vi "File Reader.vi"(0 "XML File Path":path, 11 "error in":errorcluster) -> (4 "Velocity Profiles":dbl[][][](array[numeric]), 6 "Intermediate Headings":dbl[](array[numeric]), 8 "Position Command Groups":T2(array[cluster]), 10 "Time Command Groups":T1(array[cluster]), 14 "Delta Time":dbl, 15 "error out":errorcluster)   [LabVIEW 2015]
uses:
  <vilib>/regexp/Match Regular Expression.xnode
panel:
  out "Play":string[](array[string])
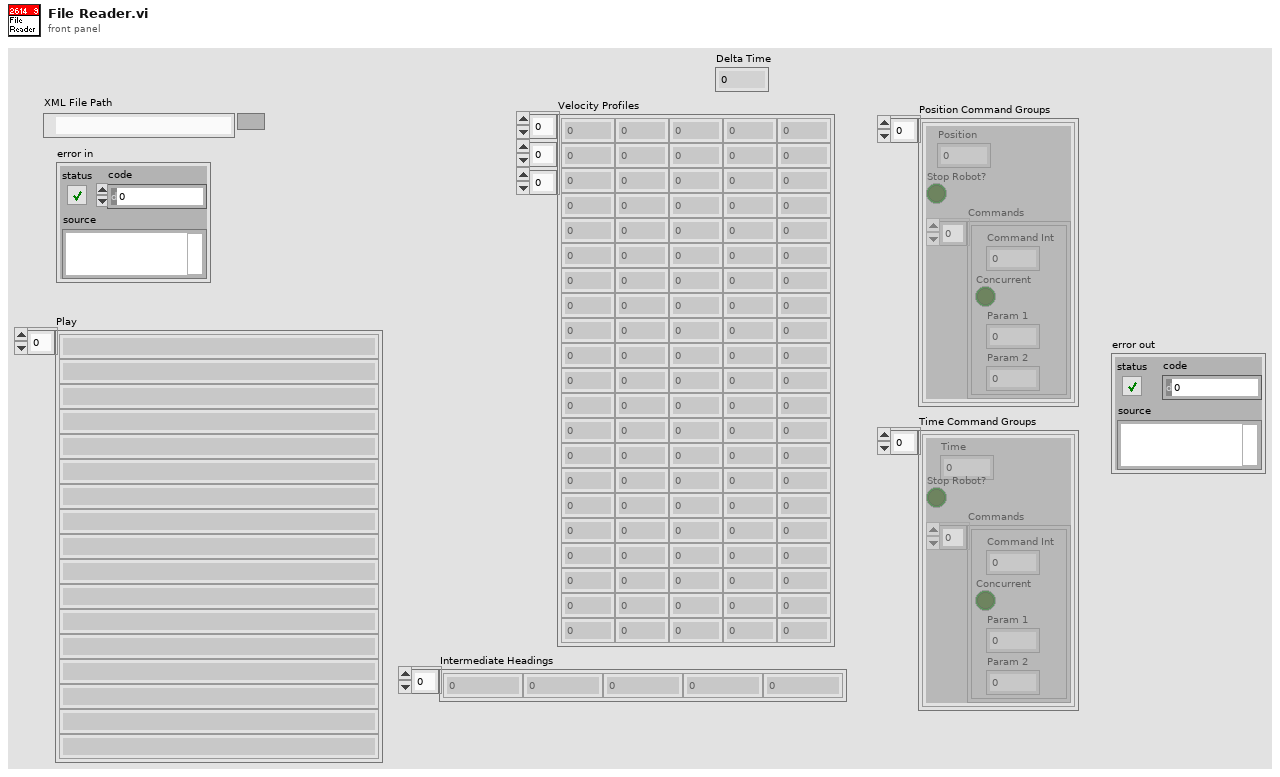
[diagram p1: front panel]
types:
  T1 = cluster{"Stop Robot?":bool, "Commands":cluster{"Command Int":i32, "Concurrent":bool, "Param 1":dbl, "Param 2":dbl}[], "Time":dbl}[]
  T2 = cluster{"Position":i32, "Stop Robot?":bool, "Commands":cluster{"Command Int":i32, "Concurrent":bool, "Param 1":dbl, "Param 2":dbl}[]}[]
  T3 = cluster{"Command Int":i32, "Concurrent":bool, "Param 1":dbl, "Param 2":dbl}[]
  T4 = cluster{"Position":i32, "Stop Robot?":bool, "Commands":cluster{"Command Int":i32, "Concurrent":bool, "Param 1":dbl, "Param 2":dbl}[]}
  T5 = cluster{"Command Int":i32, "Concurrent":bool, "Param 1":dbl, "Param 2":dbl}
  T6 = cluster{"Stop Robot?":bool, "Commands":cluster{"Command Int":i32, "Concurrent":bool, "Param 1":dbl, "Param 2":dbl}[], "Time":dbl}
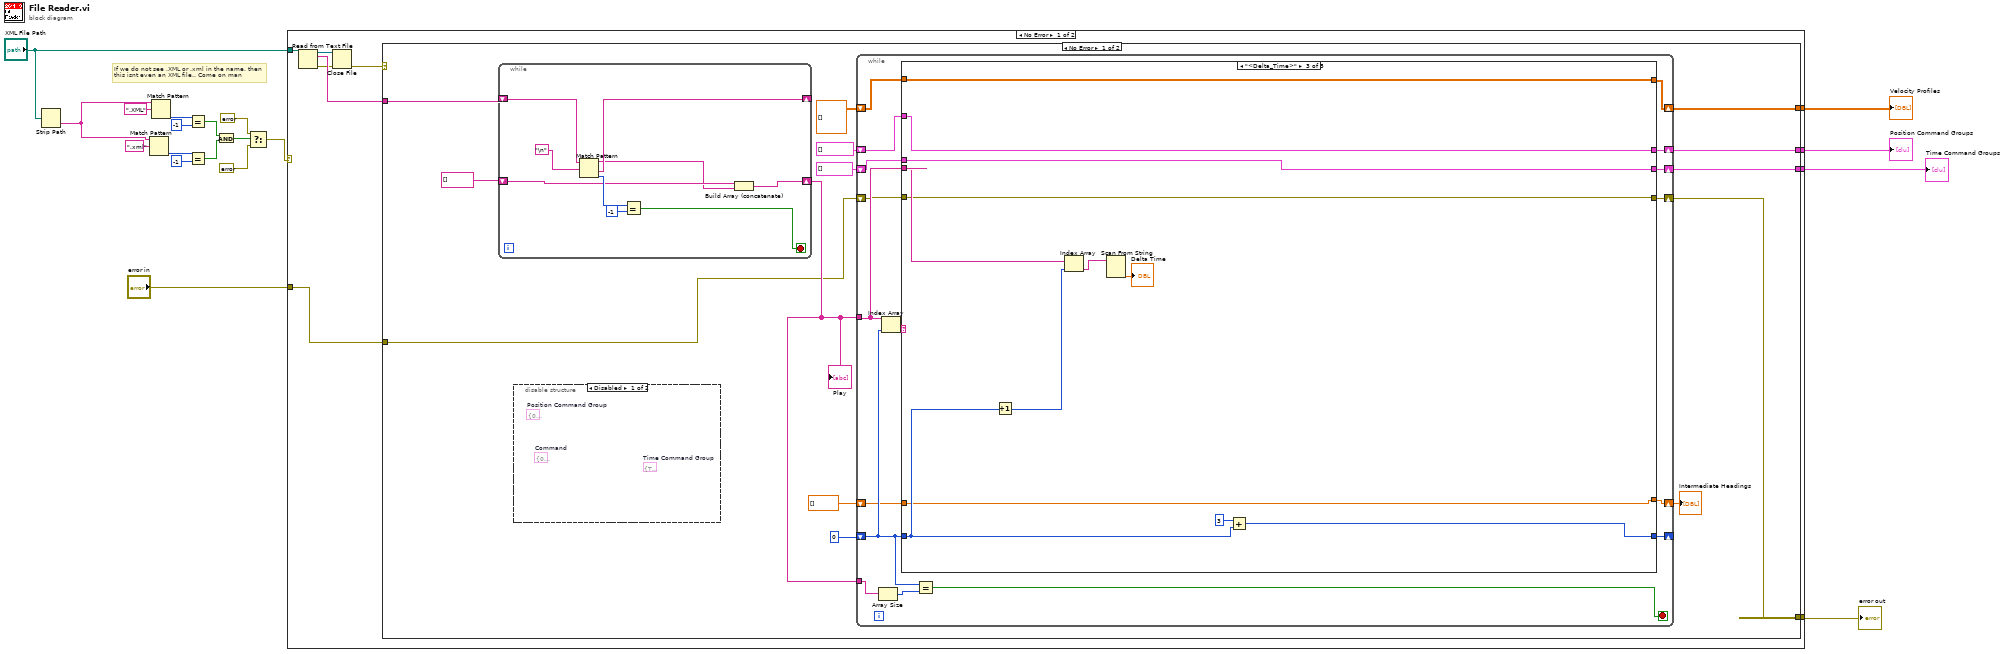
[diagram p0: block diagram]
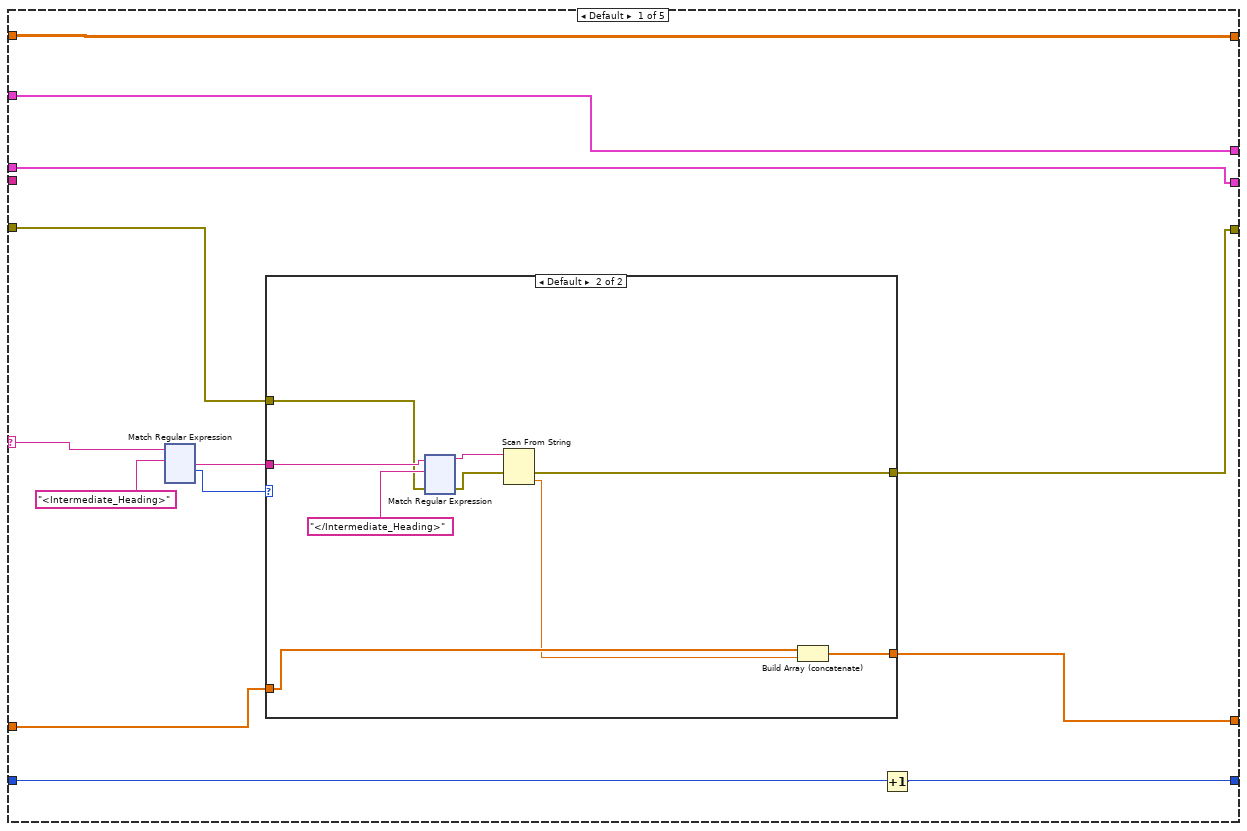
[diagram p3: hidden frame]
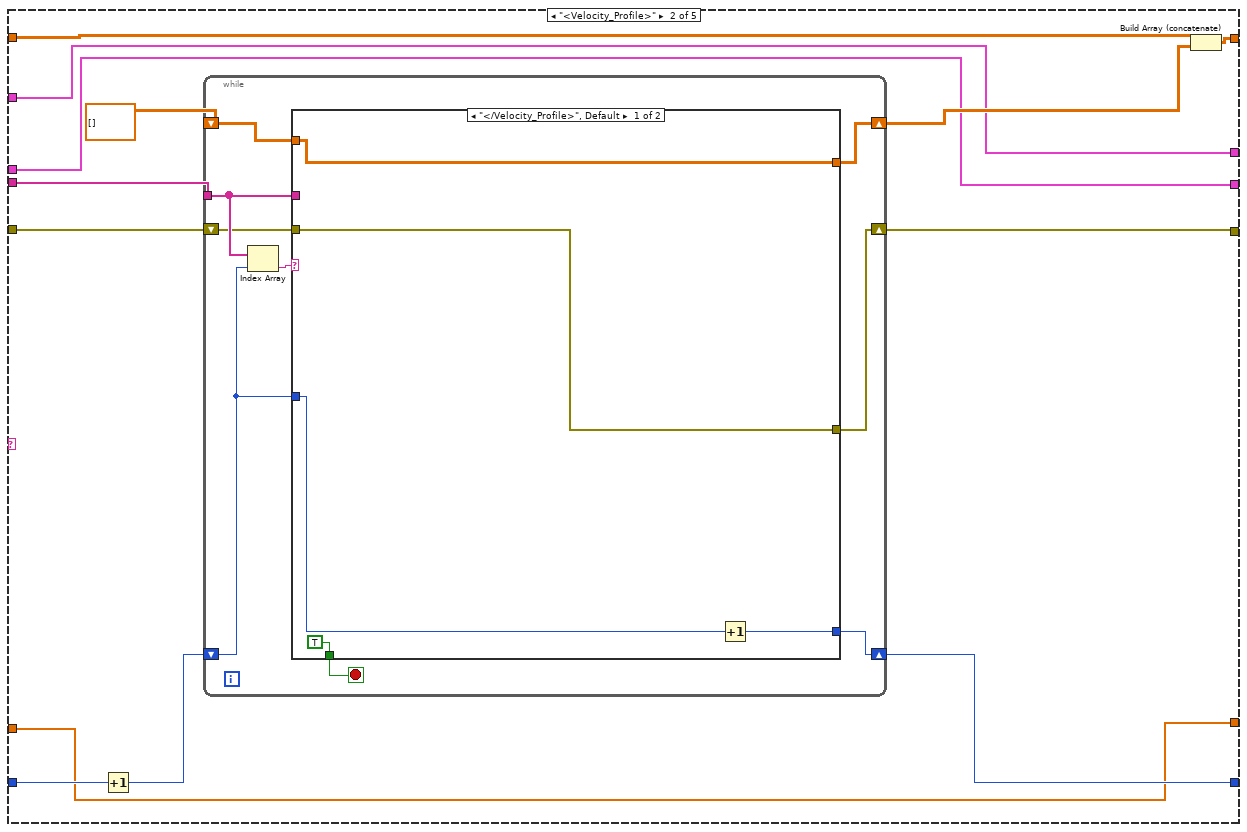
[diagram p5: hidden frame]
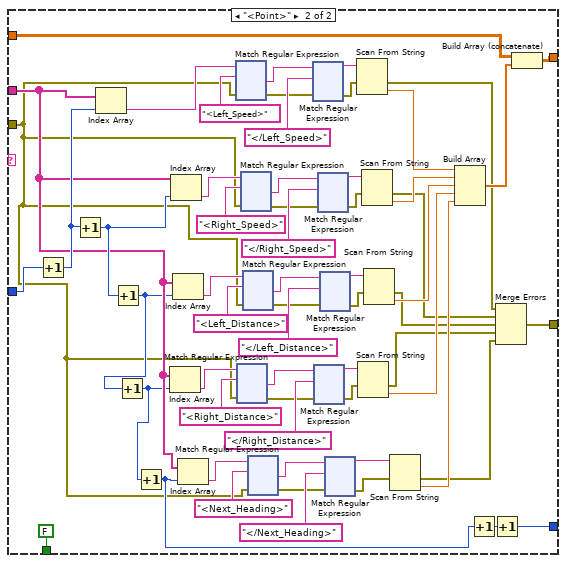
[diagram p6: hidden frame]
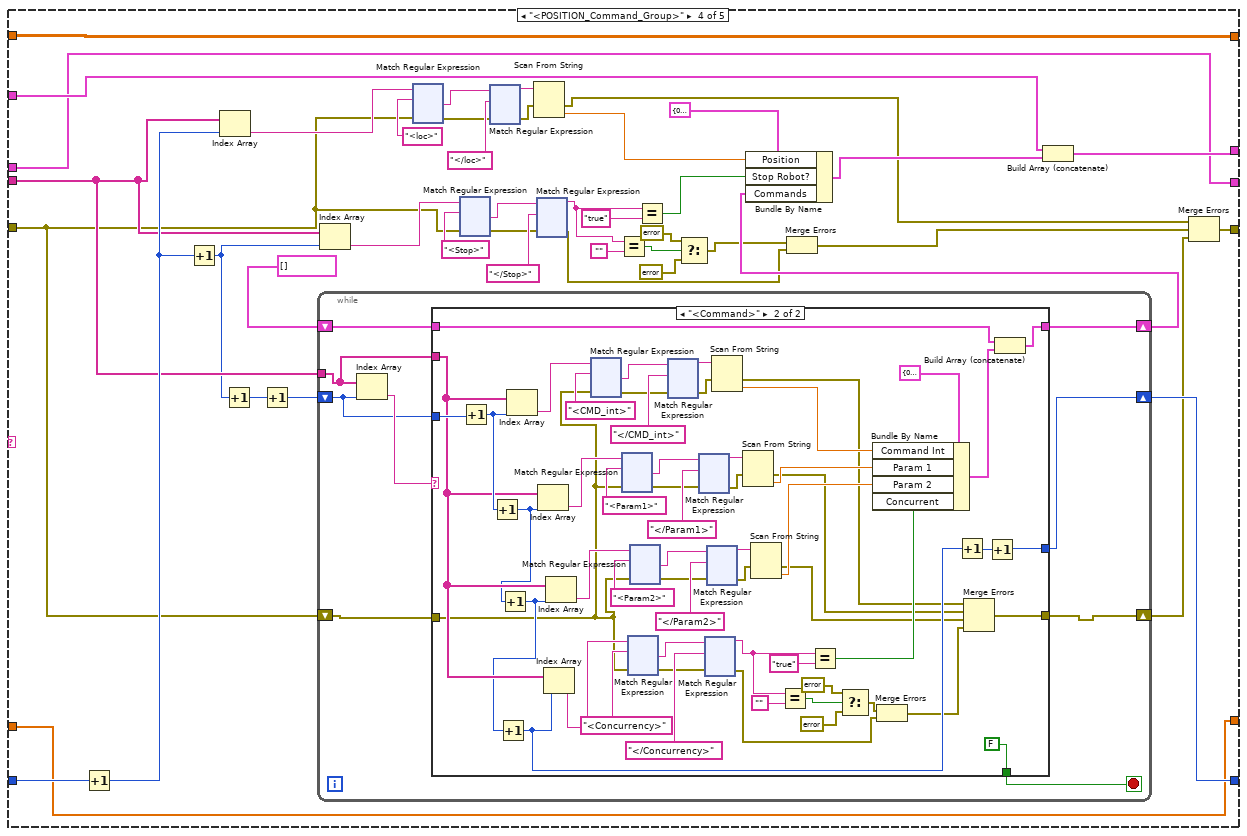
[diagram p7: hidden frame]
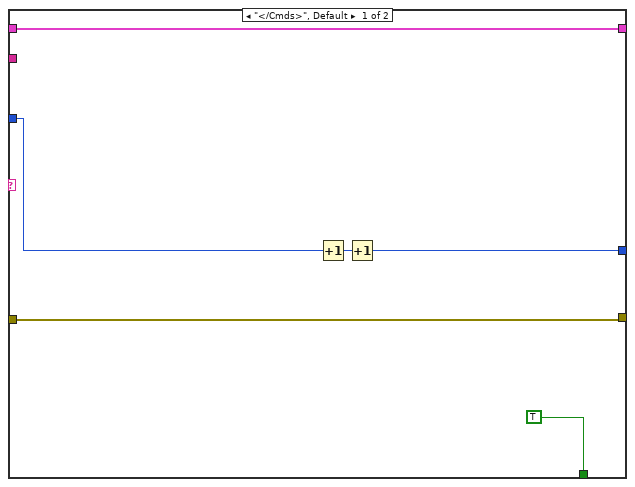
[diagram p8: hidden frame]
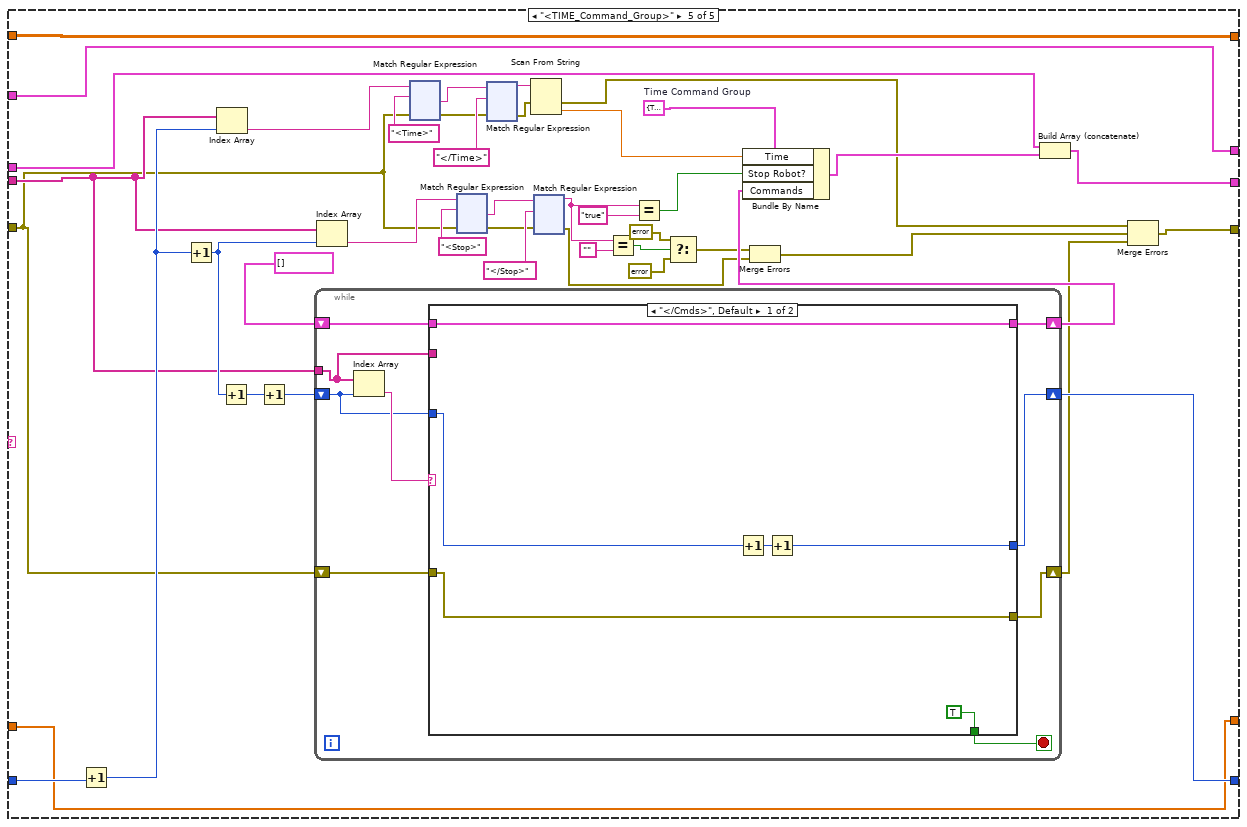
[diagram p9: hidden frame]
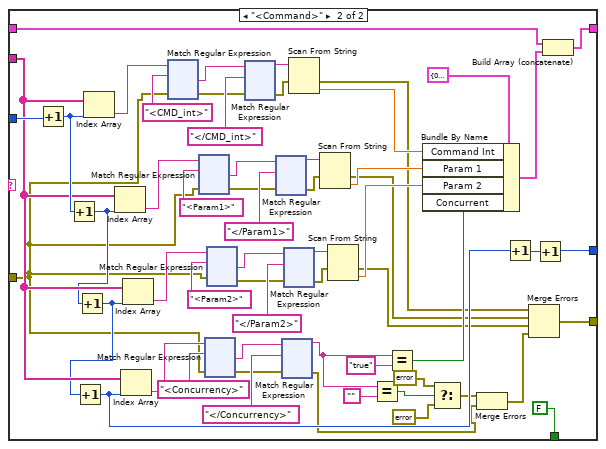
[diagram p10: hidden frame]
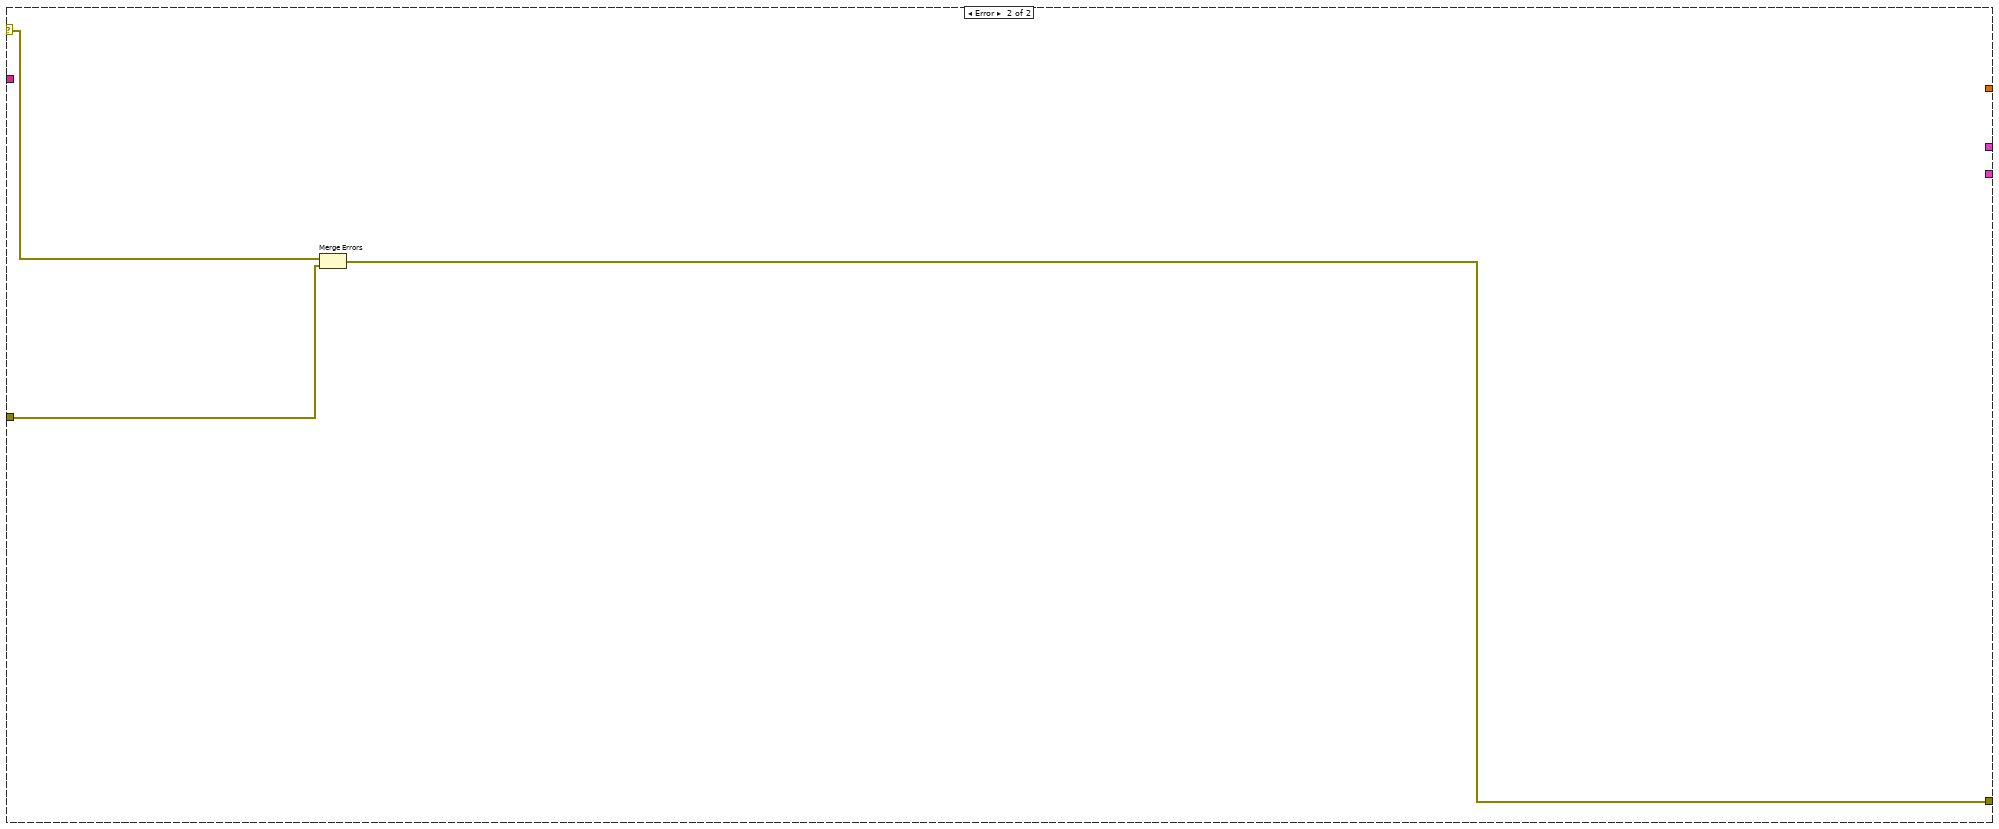
[diagram p11: hidden frame]
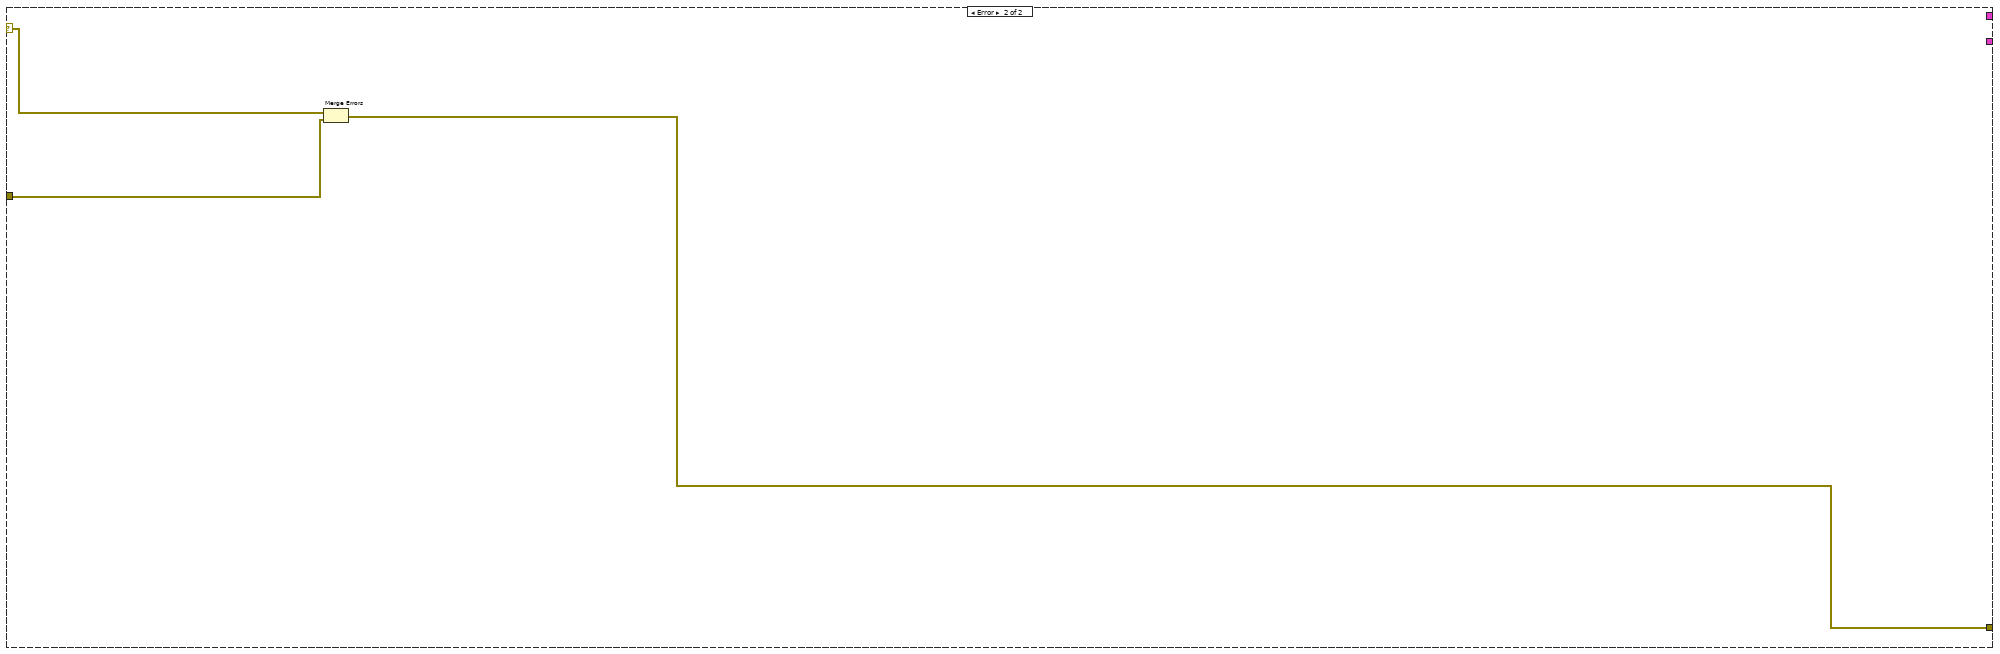
[diagram p12: hidden frame]
diagram:
  # "If we do not see .XML or .xml in the name. then\nthis isnt even an XML file.. Come on man"
  n1 = Strip Path(path="XML File Path") -> (name=w17:string)  [unwired: 1 out]
  n2 = Match Pattern(string=w17, regular expression=".xml") -> (offset past match=w13:i32)  [unwired: 1 in, 3 out]
  n3 = Match Pattern(string=w17, regular expression=".XML") -> (offset past match=w16:i32)  [unwired: 1 in, 3 out]
  n4 = Equal?(x=w16, y=-1) -> (x = y?=w12:bool)
  n5 = Equal?(x=w13, y=-1) -> (x = y?=w11:bool)
  n6 = And(x=w12, y=w11) -> (x .and. y?=w10:bool)
  n7 = Select(t=errorcluster {"status"=TRUE, "code"=13, "source"="File is not an XML File"} ("error in"), s=w10, f=errorcluster {"status"=FALSE, "code"=0, "source"=""} ("error in")) -> (s? t:f=w7:errorcluster)
  n8 = case shown="No Error" w7 {
    selector: w7 -> [_ w4532]
    tunnel: "XML File Path" -> [w29 _]
    tunnel: [w26 w4530] -> w5
    tunnel: "error in" -> [w27 w4531]
    tunnel: [w22 _] -> w3
    tunnel: [w21 _] -> w1
    tunnel: [w20 _] -> w2
    frame No Error {
      n9 = Read from Text File(file (use dialog)=w29) -> (refnum out=w24:refnum<file>, text=w28:string, error out=w25:errorcluster)  [unwired: 3 in, 1 out]
      n10 = Close File(refnum=w24, error in=w25) -> (error out=w23:errorcluster)  [unwired: 1 out]
      n11 = case shown="No Error" w23 {
        selector: w23 -> [_ w4529]
        tunnel: w28 -> [w43 _]
        tunnel: w27 -> [w34 w4528]
        tunnel: [w33 w4527] -> w26
        tunnel: [w32 _] -> w22
        tunnel: [w31 _] -> w21
        tunnel: [w30 _] -> w20
        frame No Error {
          n12 = while {
            shift-right: [w4525] -> _
            shift-left: w43 -> [w4526]
            shift-right: [w4524] -> w37
            shift-left: string[] [] -> [w4519]
            stop <- w4521 stop-if-true
            n13 = Match Pattern(string=w4526, regular expression="\n") -> (before substring=w4518:string, after substring=w4525:string, offset past match=w4523:i32)  [unwired: 1 in, 1 out]
            n14 = Equal?(x=w4523, y=-1) -> (x = y?=w4521:bool)
            n15 = Build Array (concatenate)(w4519, w4518) -> (w4524:string[])
          }
          "Play" <- w37
          n16 = disable-structure shown="Disabled" {
            frame Disabled {
              (unwired) T6 {"Stop Robot?"=TRUE, "Commands"=[], "Time"=0.0}  # Time Command Group
              (unwired) T5 {"Command Int"=0, "Concurrent"=FALSE, "Param 1"=0.0, "Param 2"=0.0}  # Command
              (unwired) T4 {"Position"=0, "Stop Robot?"=TRUE, "Commands"=[]}  # Position Command Group
            }
            frame Enabled {
            }
          }
          n17 = while {
            tunnel: w37 -> [w59]
            shift-right: [w58] -> _
            shift-left: 0 -> [w55]
            shift-right: [w56] -> w32
            shift-left: dbl[][][] [] -> [w57]
            tunnel: w37 -> [w53]
            shift-right: [w49] -> w31
            shift-left: T2 [] ("array") -> [w51]
            shift-right: [w48] -> w30
            shift-left: T1 [] ("array") -> [w50]
            shift-right: [w46] -> w35
            shift-left: dbl[] [] ("array") -> [w47]
            shift-right: [w45] -> w33
            shift-left: w34 -> [w44]
            stop <- w52 stop-if-true
            n18 = Array Size(array=w53) -> (size(s)=w54:i32)
            n19 = Index Array(array=w59, index=w55) -> (element=w60:string)
            n20 = case shown="\"<Delta_Time>\"" w60 {
              selector: w60 -> [w70 _ _ _ _]
              tunnel: w59 -> [_ w325 w1550 w1578 w3058]
              tunnel: w55 -> [w66 w324 w1544 w1586 w3057]
              tunnel: [w65 w321 w1542 w1576 w3056] -> w58
              tunnel: w57 -> [w73 w319 w1548 w1594 w3054]
              tunnel: [w73 w318 w1548 w1594 w3054] -> w56
              tunnel: w51 -> [w72 w317 w1547 w1571 w3051]
              tunnel: [w72 w317 w1547 w1570 w3051] -> w49
              tunnel: w50 -> [w71 w316 w1546 w1567 w3055]
              tunnel: [w71 w316 w1546 w1567 w3052] -> w48
              tunnel: w47 -> [w64 w315 w1541 w1568 w3050]
              tunnel: [w63 w315 w1541 w1568 w3050] -> w46
              tunnel: [w61 w313 w1545 w1553 w3040] -> w45
              tunnel: w44 -> [w62 w314 w1545 w1552 w3041]
              frame Default {
                n21 = xnode "Match Regular Expression"("input string"=w70, "regular expression"="<Intermediate_Heading>") -> ("after match"=w68:string, "offset past match"=w67:i32)  [unwired: 4 in, 3 out]
                n22 = case shown="Default" w67 {
                  tunnel: w68 -> [_ w198]
                  tunnel: w64 -> [w189 w195]
                  tunnel: [w189 w193] -> w63
                  tunnel: w62 -> [w188 w192]
                  tunnel: [w188 w190] -> w61
                  frame -1 {
                  }
                  frame Default {
                    n23 = xnode "Match Regular Expression"("input string"=w198, "regular expression"="</Intermediate_Heading>", "error in"=w192) -> ("before match"=w196:string, "error out"=w191:errorcluster)  [unwired: 3 in, 3 out]
                    n24 = Scan From String(input string=w196, error in=w191) -> (error out=w190:errorcluster, output 1=w194:dbl)  [unwired: 3 in, 2 out]
                    n25 = Build Array (concatenate)(w195, w194) -> (w193:dbl[])
                  }
                }
                n26 = Increment(x=w66) -> (x+1=w65:i32)
              }
              frame "<Velocity_Profile>" {
                n27 = Increment(x=w324) -> (x+1=w323:i32)
                n28 = while {
                  tunnel: w325 -> [w333]
                  shift-right: [w329] -> w321
                  shift-left: w323 -> [w332]
                  shift-right: [w330] -> w320
                  shift-left: dbl[][] [] -> [w331]
                  shift-right: [w326] -> w313
                  shift-left: w314 -> [w327]
                  stop <- w328 stop-if-true
                  n29 = Index Array(array=w333, index=w332) -> (element=w334:string)
                  n30 = case shown="\"</Velocity_Profile>\", Default" w334 {
                    tunnel: w333 -> [_ w364]
                    tunnel: w332 -> [w338 w399]
                    tunnel: w331 -> [w339 w371]
                    tunnel: [w339 w370] -> w330
                    tunnel: [w337 w357] -> w329
                    tunnel: [TRUE FALSE] -> w328
                    tunnel: w327 -> [w335 w356]
                    tunnel: [w335 w340] -> w326
                    frame "</Velocity_Profile>", Default {
                      n31 = Increment(x=w338) -> (x+1=w337:i32)
                    }
                    frame "<Point>" {
                      n32 = Increment(x=w399) -> (x+1=w392:i32)
                      n33 = Increment(x=w392) -> (x+1=w380:i32)
                      n34 = Index Array(array=w364, index=w392) -> (element=w398:string)
                      n35 = Increment(x=w380) -> (x+1=w359:i32)
                      n36 = Increment(x=w359) -> (x+1=w358:i32)
                      n37 = Increment(x=w358) -> (x+1=w363:i32)
                      n38 = Index Array(array=w364, index=w358) -> (element=w374:string)
                      n39 = Index Array(array=w364, index=w380) -> (element=w387:string)
                      n40 = Index Array(array=w364, index=w359) -> (element=w385:string)
                      n41 = Index Array(array=w364, index=w363) -> (element=w366:string)
                      n42 = xnode "Match Regular Expression"("input string"=w398, "regular expression"="<Left_Speed>", "error in"=w356) -> ("after match"=w396:string, "error out"=w347:errorcluster)  [unwired: 3 in, 3 out]
                      n43 = xnode "Match Regular Expression"("input string"=w374, "regular expression"="<Right_Distance>", "error in"=w356) -> ("after match"=w376:string, "error out"=w352:errorcluster)  [unwired: 3 in, 3 out]
                      n44 = xnode "Match Regular Expression"("input string"=w387, "regular expression"="<Right_Speed>", "error in"=w356) -> ("after match"=w389:string, "error out"=w348:errorcluster)  [unwired: 3 in, 3 out]
                      n45 = xnode "Match Regular Expression"("input string"=w385, "regular expression"="<Left_Distance>", "error in"=w356) -> ("after match"=w383:string, "error out"=w351:errorcluster)  [unwired: 3 in, 3 out]
                      n46 = xnode "Match Regular Expression"("input string"=w366, "regular expression"="<Next_Heading>", "error in"=w356) -> ("after match"=w368:string, "error out"=w355:errorcluster)  [unwired: 3 in, 3 out]
                      n47 = xnode "Match Regular Expression"("input string"=w396, "regular expression"="</Left_Speed>", "error in"=w347) -> ("before match"=w395:string, "error out"=w346:errorcluster)  [unwired: 3 in, 3 out]
                      n48 = xnode "Match Regular Expression"("input string"=w376, "regular expression"="</Right_Distance>", "error in"=w352) -> ("before match"=w377:string, "error out"=w353:errorcluster)  [unwired: 3 in, 3 out]
                      n49 = xnode "Match Regular Expression"("input string"=w389, "regular expression"="</Right_Speed>", "error in"=w348) -> ("before match"=w390:string, "error out"=w349:errorcluster)  [unwired: 3 in, 3 out]
                      n50 = xnode "Match Regular Expression"("input string"=w383, "regular expression"="</Left_Distance>", "error in"=w351) -> ("before match"=w382:string, "error out"=w350:errorcluster)  [unwired: 3 in, 3 out]
                      n51 = xnode "Match Regular Expression"("input string"=w368, "regular expression"="</Next_Heading>", "error in"=w355) -> ("before match"=w360:string, "error out"=w354:errorcluster)  [unwired: 3 in, 3 out]
                      n52 = Scan From String(input string=w395, error in=w346) -> (error out=w341:errorcluster, output 1=w393:dbl)  [unwired: 3 in, 2 out]
                      n53 = Scan From String(input string=w377, error in=w353) -> (error out=w344:errorcluster, output 1=w373:dbl)  [unwired: 3 in, 2 out]
                      n54 = Scan From String(input string=w390, error in=w349) -> (error out=w342:errorcluster, output 1=w386:dbl)  [unwired: 3 in, 2 out]
                      n55 = Scan From String(input string=w382, error in=w350) -> (error out=w343:errorcluster, output 1=w379:dbl)  [unwired: 3 in, 2 out]
                      n56 = Scan From String(input string=w360, error in=w354) -> (error out=w345:errorcluster, output 1=w365:dbl)  [unwired: 3 in, 2 out]
                      n57 = Build Array(w393, w386, w379, w373, w365) -> (w372:dbl[])
                      n58 = Increment(x=w363) -> (x+1=w362:i32)
                      n59 = Increment(x=w362) -> (x+1=w357:i32)
                      n60 = Merge Errors(w341, w342, w343, w344, w345) -> (w340:errorcluster)
                      n61 = Build Array (concatenate)(w371, w372) -> (w370:dbl[][])
                    }
                  }
                }
                n62 = Build Array (concatenate)(w319, w320) -> (w318:dbl[][][])
              }
              frame "<Delta_Time>" {
                n63 = Increment(x=w1544) -> (x+1=w1551:i32)
                n64 = Index Array(array=w1550, index=w1551) -> (element=w1549:string)
                n65 = Scan From String(input string=w1549) -> (output 1=→"Delta Time":dbl)  [unwired: 4 in, 3 out]
                n66 = Add(x=3, y=w1544) -> (x+y=w1542:i32)
              }
              frame "<POSITION_Command_Group>" {
                n67 = Increment(x=w1586) -> (x+1=w1579:i32)
                n68 = Increment(x=w1579) -> (x+1=w1577:i32)
                n69 = Index Array(array=w1578, index=w1579) -> (element=w1593:string)
                n70 = Increment(x=w1577) -> (x+1=w1575:i32)
                n71 = Increment(x=w1575) -> (x+1=w1569:i32)
                n72 = while {
                  tunnel: w1578 -> [w1602]
                  shift-right: [w1597] -> w1576
                  shift-left: w1569 -> [w1601]
                  shift-right: [w1599] -> w1573
                  shift-left: T3 [] ("Commands") -> [w1600]
                  shift-right: [w1596] -> w1556
                  shift-left: w1552 -> [w1595]
                  stop <- w1598 stop-if-true
                  n73 = Index Array(array=w1602, index=w1601) -> (element=w1603:string)
                  n74 = case shown="\"<Command>\"" w1603 {
                    tunnel: w1602 -> [_ w1643]
                    tunnel: w1601 -> [w1607 w1661]
                    tunnel: w1600 -> [w1609 w1635]
                    tunnel: [w1609 w1634] -> w1599
                    tunnel: [TRUE FALSE] -> w1598
                    tunnel: [w1605 w1630] -> w1597
                    tunnel: [w1604 w1614] -> w1596
                    tunnel: w1595 -> [w1604 w1610]
                    frame "</Cmds>", Default {
                      n75 = Increment(x=w1607) -> (x+1=w1606:i32)
                      n76 = Increment(x=w1606) -> (x+1=w1605:i32)
                    }
                    frame "<Command>" {
                      n77 = Increment(x=w1661) -> (x+1=w1644:i32)
                      n78 = Increment(x=w1644) -> (x+1=w1642:i32)
                      n79 = Increment(x=w1642) -> (x+1=w1641:i32)
                      n80 = Increment(x=w1641) -> (x+1=w1632:i32)
                      n81 = Index Array(array=w1643, index=w1644) -> (element=w1666:string)
                      n82 = Index Array(array=w1643, index=w1642) -> (element=w1654:string)
                      n83 = Index Array(array=w1643, index=w1632) -> (element=w1645:string)
                      n84 = Index Array(array=w1643, index=w1641) -> (element=w1653:string)
                      n85 = xnode "Match Regular Expression"("input string"=w1666, "regular expression"="<CMD_int>", "error in"=w1610) -> ("after match"=w1664:string, "error out"=w1623:errorcluster)  [unwired: 3 in, 3 out]
                      n86 = xnode "Match Regular Expression"("input string"=w1654, "regular expression"="<Param1>", "error in"=w1610) -> ("after match"=w1656:string, "error out"=w1626:errorcluster)  [unwired: 3 in, 3 out]
                      n87 = xnode "Match Regular Expression"("input string"=w1645, "regular expression"="<Concurrency>", "error in"=w1610) -> ("after match"=w1647:string, "error out"=w1627:errorcluster)  [unwired: 3 in, 3 out]
                      n88 = xnode "Match Regular Expression"("input string"=w1653, "regular expression"="<Param2>", "error in"=w1610) -> ("after match"=w1651:string, "error out"=w1629:errorcluster)  [unwired: 3 in, 3 out]
                      n89 = xnode "Match Regular Expression"("input string"=w1664, "regular expression"="</CMD_int>", "error in"=w1623) -> ("before match"=w1663:string, "error out"=w1624:errorcluster)  [unwired: 3 in, 3 out]
                      n90 = xnode "Match Regular Expression"("input string"=w1656, "regular expression"="</Param1>", "error in"=w1626) -> ("before match"=w1657:string, "error out"=w1625:errorcluster)  [unwired: 3 in, 3 out]
                      n91 = xnode "Match Regular Expression"("input string"=w1647, "regular expression"="</Concurrency>", "error in"=w1627) -> ("before match"=w1622:string, "error out"=w1612:errorcluster)  [unwired: 3 in, 3 out]
                      n92 = xnode "Match Regular Expression"("input string"=w1651, "regular expression"="</Param2>", "error in"=w1629) -> ("before match"=w1650:string, "error out"=w1628:errorcluster)  [unwired: 3 in, 3 out]
                      n93 = Scan From String(input string=w1663, error in=w1624) -> (error out=w1617:errorcluster, output 1=w1659:dbl)  [unwired: 3 in, 2 out]
                      n94 = Scan From String(input string=w1657, error in=w1625) -> (error out=w1616:errorcluster, output 1=w1637:dbl)  [unwired: 3 in, 2 out]
                      n95 = Scan From String(input string=w1650, error in=w1628) -> (error out=w1615:errorcluster, output 1=w1638:dbl)  [unwired: 3 in, 2 out]
                      n96 = Equal?(x=w1622, y="") -> (x = y?=w1618:bool)
                      n97 = Equal?(x=w1622, y="true") -> (x = y?=w1639:bool)
                      n98 = Select(t=errorcluster {"status"=TRUE, "code"=1, "source"="Scan Failed"} ("error IO"), s=w1618, f=errorcluster {"status"=FALSE, "code"=0, "source"=""} ("error IO")) -> (s? t:f=w1613:errorcluster)
                      n99 = Bundle By Name(cluster=T5 {"Command Int"=0, "Concurrent"=FALSE, "Param 1"=0.0, "Param 2"=0.0} ("Command"), "Command Int"=w1659, "Param 1"=w1637, "Param 2"=w1638, "Concurrent"=w1639) -> (w1636:T5)
                      n100 = Merge Errors(w1613, w1612) -> (w1611:errorcluster)
                      n101 = Increment(x=w1632) -> (x+1=w1631:i32)
                      n102 = Merge Errors(w1617, w1616, w1615, w1611) -> (w1614:errorcluster)
                      n103 = Increment(x=w1631) -> (x+1=w1630:i32)
                      n104 = Build Array (concatenate)(w1635, w1636) -> (w1634:T3)
                    }
                  }
                }
                n105 = Index Array(array=w1578, index=w1577) -> (element=w1585:string)
                n106 = xnode "Match Regular Expression"("input string"=w1593, "regular expression"="<loc>", "error in"=w1552) -> ("after match"=w1591:string, "error out"=w1566:errorcluster)  [unwired: 3 in, 3 out]
                n107 = xnode "Match Regular Expression"("input string"=w1585, "regular expression"="<Stop>", "error in"=w1552) -> ("after match"=w1583:string, "error out"=w1564:errorcluster)  [unwired: 3 in, 3 out]
                n108 = xnode "Match Regular Expression"("input string"=w1591, "regular expression"="</loc>", "error in"=w1566) -> ("before match"=w1590:string, "error out"=w1565:errorcluster)  [unwired: 3 in, 3 out]
                n109 = Scan From String(input string=w1590, error in=w1565) -> (error out=w1554:errorcluster, output 1=w1587:dbl)  [unwired: 3 in, 2 out]
                n110 = xnode "Match Regular Expression"("input string"=w1583, "regular expression"="</Stop>", "error in"=w1564) -> ("before match"=w1559:string, "error out"=w1558:errorcluster)  [unwired: 3 in, 3 out]
                n111 = Equal?(x=w1559, y="") -> (x = y?=w1560:bool)
                n112 = Equal?(x=w1559, y="true") -> (x = y?=w1580:bool)
                n113 = Select(t=errorcluster {"status"=TRUE, "code"=1, "source"="Scan Failed"} ("error IO"), s=w1560, f=errorcluster {"status"=FALSE, "code"=0, "source"=""} ("error IO")) -> (s? t:f=w1557:errorcluster)
                n114 = Bundle By Name(cluster=T4 {"Position"=0, "Stop Robot?"=TRUE, "Commands"=[]} ("Position Command Group"), "Position"=w1587, "Stop Robot?"=w1580, "Commands"=w1573) -> (w1572:T4)
                n115 = Merge Errors(w1557, w1558) -> (w1555:errorcluster)
                n116 = Build Array (concatenate)(w1571, w1572) -> (w1570:T2)
                n117 = Merge Errors(w1554, w1555, w1556) -> (w1553:errorcluster)
              }
              frame "<TIME_Command_Group>" {
                w3053 = T6 {"Stop Robot?"=TRUE, "Commands"=[], "Time"=0.0}  # Time Command Group
                n118 = Increment(x=w3057) -> (x+1=w3065:i32)
                n119 = Increment(x=w3065) -> (x+1=w3064:i32)
                n120 = Index Array(array=w3058, index=w3065) -> (element=w3077:string)
                n121 = Increment(x=w3064) -> (x+1=w3063:i32)
                n122 = Increment(x=w3063) -> (x+1=w3059:i32)
                n123 = while {
                  tunnel: w3058 -> [w3085]
                  shift-right: [w3080] -> w3056
                  shift-left: w3059 -> [w3084]
                  shift-right: [w3082] -> w3061
                  shift-left: T3 [] ("Commands") -> [w3083]
                  shift-right: [w3078] -> w3039
                  shift-left: w3041 -> [w3079]
                  stop <- w3081 stop-if-true
                  n124 = Index Array(array=w3085, index=w3084) -> (element=w3086:string)
                  n125 = case shown="\"</Cmds>\", Default" w3086 {
                    tunnel: w3085 -> [_ w3126]
                    tunnel: w3084 -> [w3090 w3144]
                    tunnel: w3083 -> [w3092 w3118]
                    tunnel: [w3092 w3117] -> w3082
                    tunnel: [TRUE FALSE] -> w3081
                    tunnel: [w3088 w3114] -> w3080
                    tunnel: w3079 -> [w3087 w3107]
                    tunnel: [w3087 w3093] -> w3078
                    frame "</Cmds>", Default {
                      n126 = Increment(x=w3090) -> (x+1=w3089:i32)
                      n127 = Increment(x=w3089) -> (x+1=w3088:i32)
                    }
                    frame "<Command>" {
                      n128 = Increment(x=w3144) -> (x+1=w3127:i32)
                      n129 = Increment(x=w3127) -> (x+1=w3125:i32)
                      n130 = Increment(x=w3125) -> (x+1=w3124:i32)
                      n131 = Increment(x=w3124) -> (x+1=w3113:i32)
                      n132 = Index Array(array=w3126, index=w3127) -> (element=w3149:string)
                      n133 = Index Array(array=w3126, index=w3125) -> (element=w3137:string)
                      n134 = Index Array(array=w3126, index=w3113) -> (element=w3128:string)
                      n135 = Index Array(array=w3126, index=w3124) -> (element=w3136:string)
                      n136 = xnode "Match Regular Expression"("input string"=w3149, "regular expression"="<CMD_int>", "error in"=w3107) -> ("after match"=w3147:string, "error out"=w3104:errorcluster)  [unwired: 3 in, 3 out]
                      n137 = xnode "Match Regular Expression"("input string"=w3137, "regular expression"="<Param1>", "error in"=w3107) -> ("after match"=w3139:string, "error out"=w3105:errorcluster)  [unwired: 3 in, 3 out]
                      n138 = xnode "Match Regular Expression"("input string"=w3128, "regular expression"="<Concurrency>", "error in"=w3107) -> ("after match"=w3130:string, "error out"=w3100:errorcluster)  [unwired: 3 in, 3 out]
                      n139 = xnode "Match Regular Expression"("input string"=w3136, "regular expression"="<Param2>", "error in"=w3107) -> ("after match"=w3134:string, "error out"=w3106:errorcluster)  [unwired: 3 in, 3 out]
                      n140 = xnode "Match Regular Expression"("input string"=w3147, "regular expression"="</CMD_int>", "error in"=w3104) -> ("before match"=w3146:string, "error out"=w3103:errorcluster)  [unwired: 3 in, 3 out]
                      n141 = xnode "Match Regular Expression"("input string"=w3139, "regular expression"="</Param1>", "error in"=w3105) -> ("before match"=w3140:string, "error out"=w3102:errorcluster)  [unwired: 3 in, 3 out]
                      n142 = xnode "Match Regular Expression"("input string"=w3130, "regular expression"="</Concurrency>", "error in"=w3100) -> ("before match"=w3108:string, "error out"=w3098:errorcluster)  [unwired: 3 in, 3 out]
                      n143 = xnode "Match Regular Expression"("input string"=w3134, "regular expression"="</Param2>", "error in"=w3106) -> ("before match"=w3133:string, "error out"=w3101:errorcluster)  [unwired: 3 in, 3 out]
                      n144 = Scan From String(input string=w3146, error in=w3103) -> (error out=w3094:errorcluster, output 1=w3142:dbl)  [unwired: 3 in, 2 out]
                      n145 = Scan From String(input string=w3140, error in=w3102) -> (error out=w3095:errorcluster, output 1=w3120:dbl)  [unwired: 3 in, 2 out]
                      n146 = Scan From String(input string=w3133, error in=w3101) -> (error out=w3096:errorcluster, output 1=w3121:dbl)  [unwired: 3 in, 2 out]
                      n147 = Equal?(x=w3108, y="") -> (x = y?=w3109:bool)
                      n148 = Equal?(x=w3108, y="true") -> (x = y?=w3122:bool)
                      n149 = Bundle By Name(cluster=T5 {"Command Int"=0, "Concurrent"=FALSE, "Param 1"=0.0, "Param 2"=0.0} ("Command"), "Command Int"=w3142, "Param 1"=w3120, "Param 2"=w3121, "Concurrent"=w3122) -> (w3119:T5)
                      n150 = Select(t=errorcluster {"status"=TRUE, "code"=1, "source"="Scan Failed"} ("error IO"), s=w3109, f=errorcluster {"status"=FALSE, "code"=0, "source"=""} ("error IO")) -> (s? t:f=w3099:errorcluster)
                      n151 = Merge Errors(w3099, w3098) -> (w3097:errorcluster)
                      n152 = Increment(x=w3113) -> (x+1=w3115:i32)
                      n153 = Merge Errors(w3094, w3095, w3096, w3097) -> (w3093:errorcluster)
                      n154 = Increment(x=w3115) -> (x+1=w3114:i32)
                      n155 = Build Array (concatenate)(w3118, w3119) -> (w3117:T3)
                    }
                  }
                }
                n156 = Index Array(array=w3058, index=w3064) -> (element=w3071:string)
                n157 = xnode "Match Regular Expression"("input string"=w3077, "regular expression"="<Time>", "error in"=w3041) -> ("after match"=w3075:string, "error out"=w3049:errorcluster)  [unwired: 3 in, 3 out]
                n158 = xnode "Match Regular Expression"("input string"=w3071, "regular expression"="<Stop>", "error in"=w3041) -> ("after match"=w3069:string, "error out"=w3047:errorcluster)  [unwired: 3 in, 3 out]
                n159 = xnode "Match Regular Expression"("input string"=w3075, "regular expression"="</Time>", "error in"=w3049) -> ("before match"=w3074:string, "error out"=w3048:errorcluster)  [unwired: 3 in, 3 out]
                n160 = Scan From String(input string=w3074, error in=w3048) -> (error out=w3036:errorcluster, output 1=w3072:dbl)  [unwired: 3 in, 2 out]
                n161 = xnode "Match Regular Expression"("input string"=w3069, "regular expression"="</Stop>", "error in"=w3047) -> ("before match"=w3042:string, "error out"=w3037:errorcluster)  [unwired: 3 in, 3 out]
                n162 = Equal?(x=w3042, y="") -> (x = y?=w3043:bool)
                n163 = Equal?(x=w3042, y="true") -> (x = y?=w3066:bool)
                n164 = Select(t=errorcluster {"status"=TRUE, "code"=1, "source"="Scan Failed"} ("error IO"), s=w3043, f=errorcluster {"status"=FALSE, "code"=0, "source"=""} ("error IO")) -> (s? t:f=w3038:errorcluster)
                n165 = Bundle By Name(cluster=w3053, "Time"=w3072, "Stop Robot?"=w3066, "Commands"=w3061) -> (w3060:T6)
                n166 = Merge Errors(w3038, w3037) -> (w3035:errorcluster)
                n167 = Build Array (concatenate)(w3055, w3060) -> (w3052:T1)
                n168 = Merge Errors(w3036, w3035, w3039) -> (w3040:errorcluster)
              }
            }
            n169 = Equal?(x=w55, y=w54) -> (x = y?=w52:bool)
          }
          "Intermediate Headings" <- w35
        }
        frame Error {
          n170 = Merge Errors(w4529, w4528) -> (w4527:errorcluster)
        }
      }
    }
    frame Error {
      n171 = Merge Errors(w4532, w4531) -> (w4530:errorcluster)
    }
  }
  "error out" <- w5
  "Velocity Profiles" <- w3
  "Position Command Groups" <- w1
  "Time Command Groups" <- w2
